vi "Time Period To Num Samples.vi"(1 "Duration (ms)":dbl, 2 "Sampling rate (Hz)":dbl) -> (6 "Samples":i32)   [LabVIEW 2020]
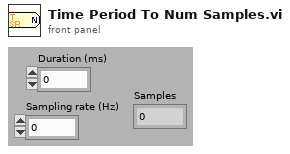
[diagram p1: front panel]
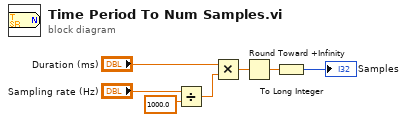
[diagram p0: block diagram]
diagram:
  n1 = Divide(x="Sampling rate (Hz)", y=1000.0) -> (x/y=w6:dbl)
  n2 = Multiply(x="Duration (ms)", y=w6) -> (x*y=w4:dbl)
  n3 = Round Toward +Infinity(x=w4) -> (ceil(x): smallest int >= x=w3:dbl)
  n4 = To Long Integer(number=w3) -> (32bit integer=→"Samples":i32)
